vi "AttackerAimGoalTactic.vi"(6 "States in":T1=enum."AimGoal", 8 "error in (no error)":errorcluster, 9 "Game in":refnum<class "Game.lvclass">, 10 "Robot":refnum<class "Robot.lvclass">, 11 "AttackerAimGoalTactic in":refnum<class "AttackerAimGoalTactic.lvclass">) -> (0 "error out":errorcluster, 2 "Robot out":refnum<class "Robot.lvclass">, 3 "AttackerAimGoalTactic out":refnum<class "AttackerAimGoalTactic.lvclass">)   [LabVIEW 2018, in "AttackerAimGoalTactic.lvclass"]
uses:
  AttackerAimGoalTactic.lvclass
  Game_class/Game.lvclass
  Robot_class/Robot.lvclass
  C:/Users/lucas/Documents/RoboIME/SSL_AI - pass/Object_class/Object.lvclass
  C:/Users/lucas/Documents/RoboIME/SSL_AI - pass/Tactic_class/Tactic.lvclass
  States.ctl
  Tactic_class/Tactic.lvclass/Tactic.ctl
  Skillbook_class/Skillbook.lvclass/Skillbook.ctl
  Game_class/Game.lvclass/Game.ctl
  Parameters_class/Parameters.lvclass/Parameters.ctl
  Object_class/Object.lvclass/Object.ctl
  Robot_class/Robot.lvclass/Robot.ctl
  AttackerAimGoalTactic.lvclass/AttackerAimGoalTactic.ctl
  <vilib>/Analysis/_algsub.llb/Real Vector Norm.vi
  Game_class/Read Parameters.lvclass.vi
  Parameters_class/Read AttakingOurselves.vi
  Skillbook_class/Read AttackerAimGoalSkill.vi
  Object_class/Read x.vi
  Object_class/Read y.vi
  Robot_class/Read orientation.vi
  Robot_class/Read dest_x.vi
  Robot_class/Read dest_y.vi
  Robot_class/Read dest_orientation.vi
  Tactic_class/Read Skillbook.vi
  Write States.vi
  Skillbook_class/Skillbook.lvclass
  Parameters_class/Parameters.lvclass
  AttackerAimGoalSkill_class/AttackerAimGoalSkill.lvclass
  <vilib>/Analysis/NI_AALPro.lvlib
panel:
  out "x .or. y?":bool
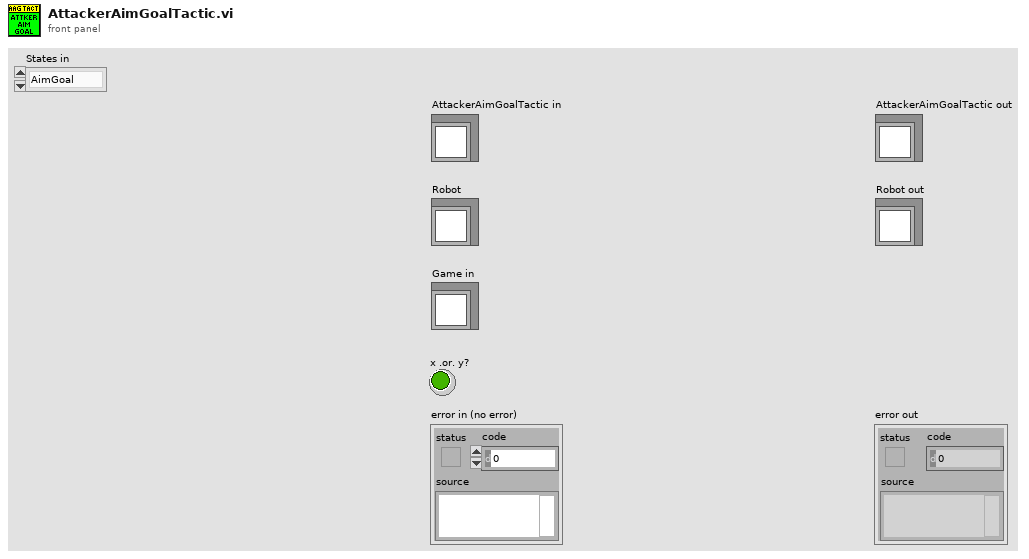
[diagram p1: front panel]
types:
  T1 = typedef "AttackerAimGoalTactic.lvclass/States.ctl" = enum16{"Exit", "AimGoal"}
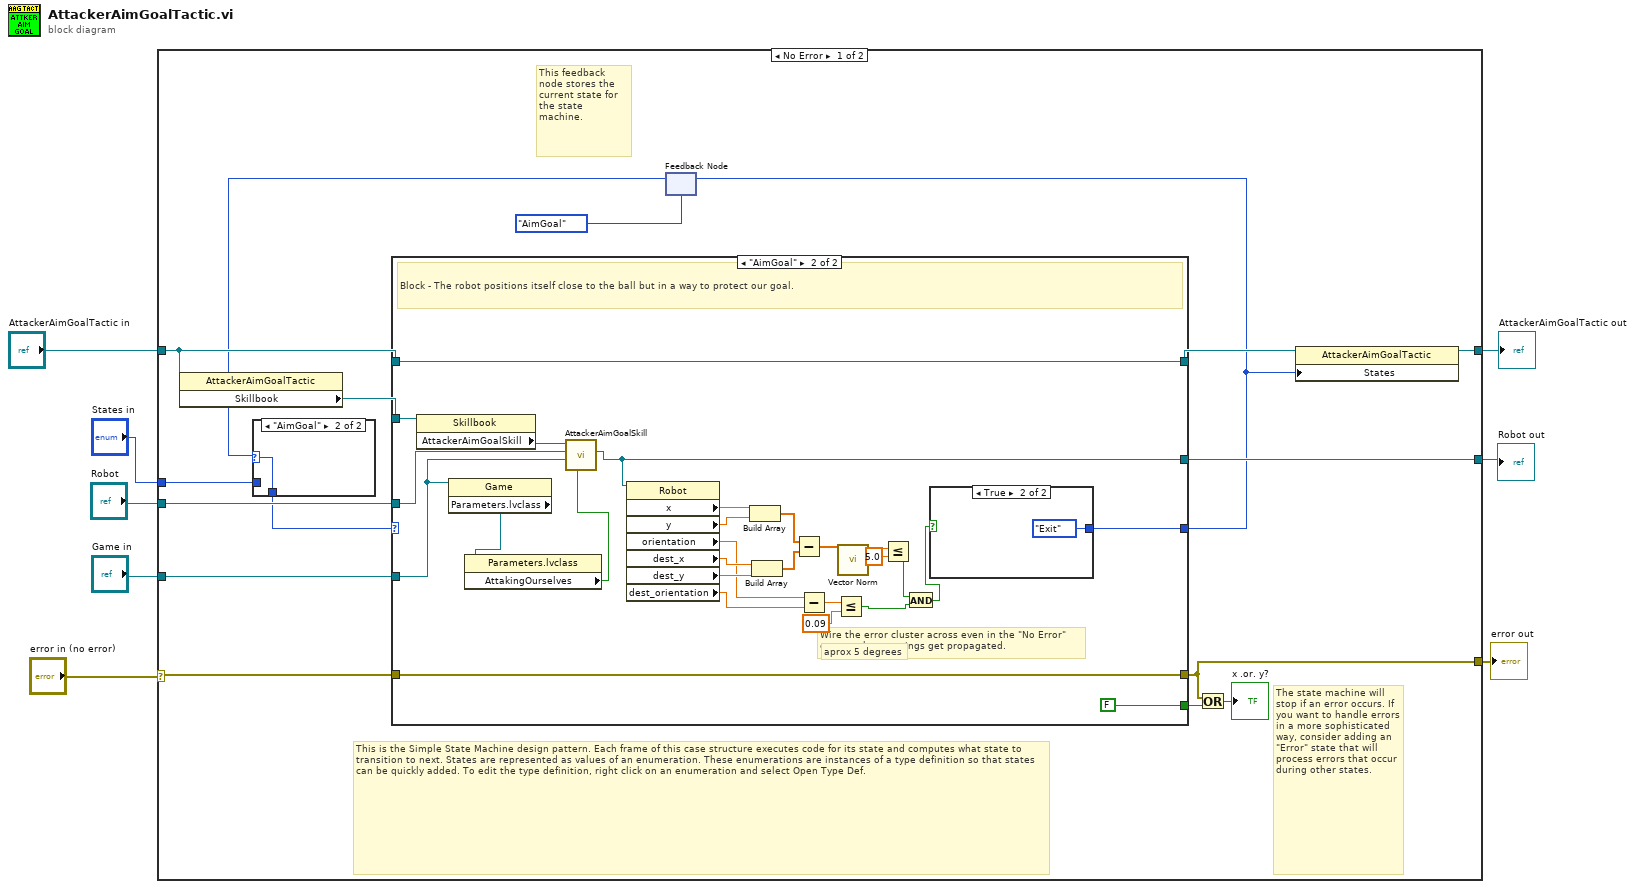
[diagram p0: block diagram]
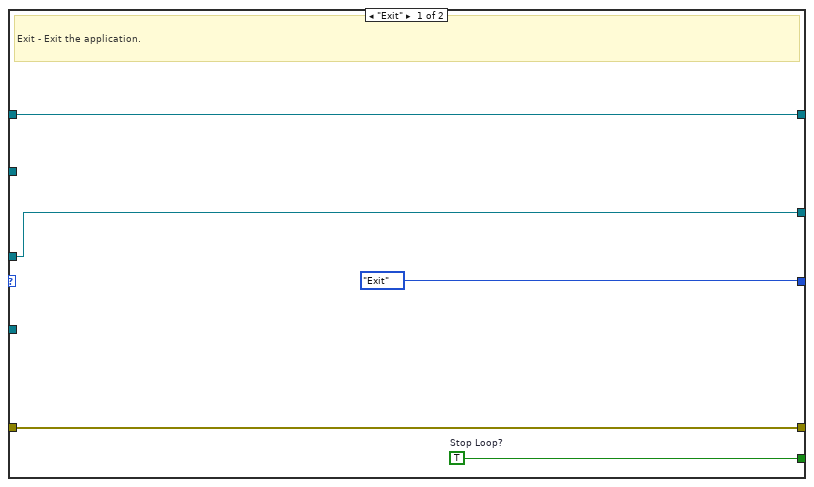
[diagram p3: hidden frame]
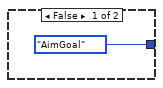
[diagram p4: hidden frame]
diagram:
  n1 = case shown="No Error" "error in (no error)" {
    selector: "error in (no error)" -> [w19 w63]
    tunnel: [w16 w63] -> w7
    tunnel: [w14 w62] -> w6
    tunnel: "AttackerAimGoalTactic in" -> [w20 w62]
    tunnel: "Robot" -> [w18 w61]
    tunnel: "Game in" -> [w17 _]
    tunnel: [w15 w61] -> w2
    tunnel: "States in" -> [w9 _]
    frame No Error {
      # "The state machine will stop if an error occurs. If you want to handle errors in a more sophisticated way, consider adding an \"Error\" state that will process errors that occur during other states."
      # "This feedback node stores the current state for the state machine."
      # "This is the Simple State Machine design pattern. Each frame of this case structure executes code for its state and computes what state to transition to next. States are represented as values of an enumeration. These enumerations are instances of a type definition so that states can be quickly added. To edit the type definition, right click on an enumeration and select Open Type Def."
      # "Wire the error cluster across even in the \"No Error\"\ncase so that warnings get propagated."
      n2 = property class="AttackerAimGoalTactic"(reference=w20) -> ("Skillbook"=w22:refnum<class "Skillbook.lvclass">)  [unwired: 1 in, 2 out]
      n3 = feedback #1(States."AimGoal" ("States")) -> (w11:T1)
      n4 = case shown="\"AimGoal\"" w11 {
        selector: w11 -> [_ w26]
        tunnel: [w25 w26] -> w10
        tunnel: w9 -> [w25 _]
        frame "Exit", Default {
        }
        frame "AimGoal" {
        }
      }
      n5 = case shown="\"AimGoal\"" w10 {
        tunnel: [w31 FALSE ("Stop Loop?")] -> w24
        tunnel: w19 -> [w30 w57]
        tunnel: [w30 w57] -> w16
        tunnel: w22 -> [_ w56]
        tunnel: w18 -> [w29 w53]
        tunnel: [w29 w48] -> w15
        tunnel: [w28 w55] -> w21
        tunnel: w20 -> [w28 w55]
        tunnel: w17 -> [_ w52]
        tunnel: [States."Exit" ("States") w49] -> w12
        frame "Exit" {
          w31 = TRUE  # Stop Loop?
          # "Exit - Exit the application."
        }
        frame "AimGoal" {
          # "aprox 5 degrees"
          # "Block - The robot positions itself close to the ball but in a way to protect our goal."
          n6 = property class="Skillbook"(reference=w56) -> ("AttackerAimGoalSkill"=w54:refnum<class "AttackerAimGoalSkill.lvclass">)  [unwired: 1 in, 2 out]
          n7 = property class="Game"(reference=w52) -> ("Parameters.lvclass"=w51:refnum<class "Parameters.lvclass">)  [unwired: 1 in, 2 out]
          n8 = property class="Parameters.lvclass"(reference=w51) -> ("AttakingOurselves"=w50:bool)  [unwired: 1 in, 2 out]
          n9 = call-dynamic "AttackerAimGoalSkill.vi"("AttackOurselves"=w50, "Game"=w52, "Robot"=w53, "AttackerAimGoalSkill in"=w54) -> ("Robot out"=w48:refnum<class "Robot.lvclass">)  [unwired: 5 in, 2 out]
          n10 = property class="Robot"(reference=w48) -> ("x"=w47:dbl, "y"=w46:dbl, "orientation"=w38:dbl, "dest_x"=w45:dbl, "dest_y"=w44:dbl, "dest_orientation"=w39:dbl)  [unwired: 1 in, 2 out]
          n11 = Build Array(w47, w46) -> (w43:dbl[])
          n12 = Build Array(w45, w44) -> (w42:dbl[])
          n13 = Subtract(x=w43, y=w42) -> (x-y=w41:dbl[])
          n14 = Subtract(x=w38, y=w39) -> (x-y=w36:dbl)
          n15 = Less Or Equal?(x=w36, y=0.09) -> (x <= y?=w33:bool)
          n16 = call-poly <vilib>:"Vector Norm.vi"("Input Vector"=w41) -> ("norm"=w40:dbl)  [unwired: 9 in, 1 out]
          n17 = Less Or Equal?(x=w40, y=5.0) -> (x <= y?=w34:bool)
          n18 = And(x=w34, y=w33) -> (x .and. y?=w32:bool)
          n19 = case shown="True" w32 {
            tunnel: [States."AimGoal" ("States") States."Exit" ("States")] -> w49
            frame False {
            }
            frame True {
            }
          }
        }
      }
      n20 = feedback-in #1(w12) -> ()
      n21 = Or(x=w16, y=w24) -> (x .or. y?=→"x .or. y?":bool)
      n22 = property class="AttackerAimGoalTactic"(reference=w21, "States"=w12) -> (reference out=w14:refnum<class "AttackerAimGoalTactic.lvclass">)  [unwired: 1 in, 1 out]
    }
    frame Error {
    }
  }
  "error out" <- w7
  "AttackerAimGoalTactic out" <- w6
  "Robot out" <- w2
